vi "final_usrp_transceiver2.vi"() -> ()   [LabVIEW 2014]
uses:
  <vilib>/addons/Modulation/Analog/support/mod_Set Error Source.vi
  var_stop.vi
  <vilib>/addons/Modulation/Digital/Support/Common/Validators/mod_Generate Filter Coefficients Validate.vi
  <vilib>/addons/Modulation/Digital/General/subVIs/mod_Generate Filter Coefficients.vi
  <vilib>/measure/maspectr.llb/FFT Power Spectrum and PSD for 1 Chan (CDB).vi
  <vilib>/addons/Modulation/Digital/General/MT Apply Matched Filter (Generic).vi
  <vilib>/addons/Modulation/Digital/General/MT Align to Ideal Symbols (Generic).vi
  <instrlib>/niUSRP/niUSRP Fetch Rx Data (CDB Cluster).vi
  <instrlib>/niUSRP/niUSRP Write Tx Data (CDB Cluster).vi
  <vilib>/addons/Modulation/Digital/General/MT Apply Pulse Shaping Filter (Generic).vi
  <vilib>/addons/Modulation/niDMT.lvlib
  <vilib>/measure/NI_MAPro.lvlib
panel:
  in  "frame buffer size":i32=20
  in  "Stop":bool
  out "Frames Per Second":u32
  in  "energy threshold":dbl=-33.0 format="%#_13g"
  out "elements in frame buffer":i32
  out "valid frames":i32
  out "elements in send buffer":i32
  in  "packet size":i32=12800
  in  "Quality (0-1000)":i32=100 caption="Quality (750)"
  out "size(s) 4":i32
  out "frame num":u32
  out "length":i32[](array[numeric])
  out "start index":i32[](array[numeric])
  out "Numeric":i32
  out "size(s) 3":i32
  out "# elements in queue 2":i32
  out "size(s) 2":i32
  out "size(s)":i32[](array[numeric])
  out "image":T1(plugin-control)
  in  "Transmit power (db)":dbl
  out "found?":bool
  out "# elements in queue":i32
  out "valid?":bool
  in  "Gray code?":bool=TRUE
  in  "Modulation":enum16{"PSK", "QAM"}(ring)
  out "packet len":u32
  in  "filter length (symbols)":i32=8
  in  "filter parameter":dbl=0.5 format="%.2f"
  in  "pulse shaping filter (none)":T2(ring)=enum."Raised Cosine"
  in  "M-PSK (4)":i32=4 caption="M-ARY"
  in  "samples per symbol (16)":i32=4
  out "packet bits length":i32
  in  "number of samples":i64=40000
  out "RX coerced gain":dbl format="%#_6f"
  out "RX coerced carrier frequency":dbl=915000000.0 format="%#_6p"
  out "RX coerced IQ rate":dbl=4000000.0 format="%#_6p"
  in  "RX active antenna":string="RX2"
  in  "RX gain":dbl format="%#_6f"
  in  "RX device names":refnum<k15>="192.168.10.2"
  out "TX coerced gain":dbl format="%#_6f"
  out "TX coerced carrier frequency":dbl=915000000.0 format="%#_6p"
  out "coerced IQ rate":dbl=4000000.0 format="%#_6p"
  in  "TX device names":refnum<k15>="192.168.10.2"
  in  "TX gain":dbl format="%#_6f"
  in  "carrier frequency":dbl=915000000.0 format="%#_6p"
  in  "IQ rate":dbl=800000.0 format="%#_6p"
  in  "stop":bool
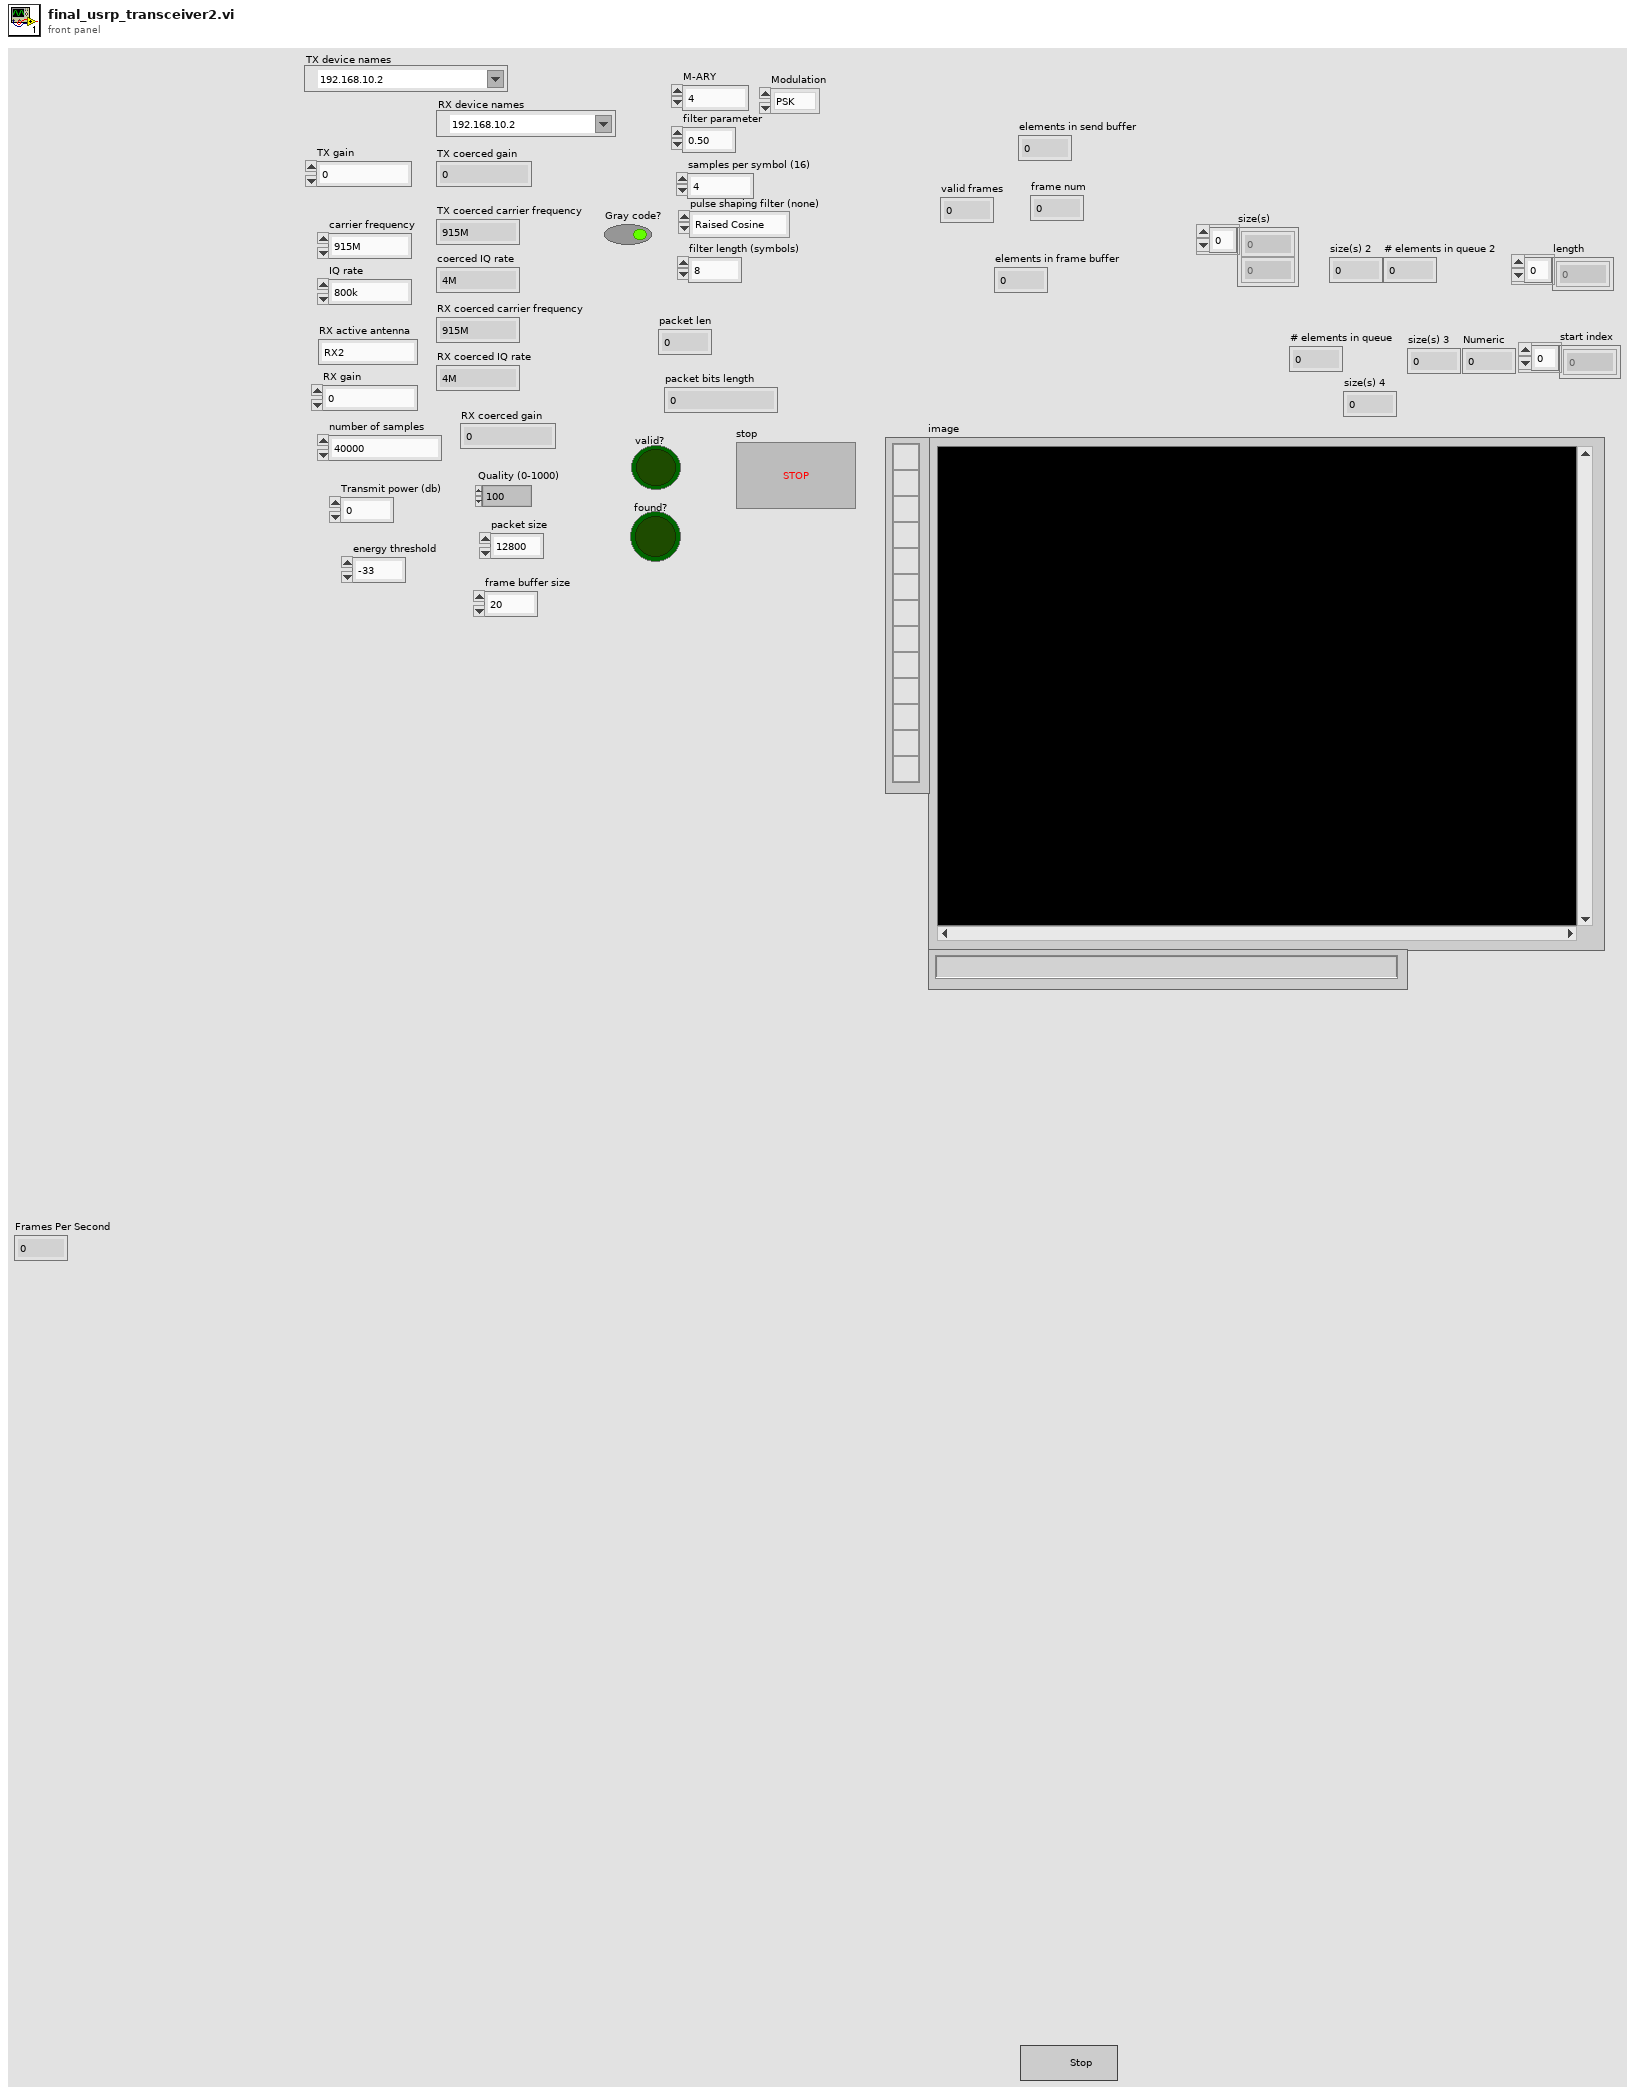
[diagram p1: front panel]
types:
  T1 = typedef "IMAQ Image.ctl" = refnum<image>
  T2 = enum16{"none", "Raised Cosine", "Root Raised Cos", "Gaussian"}
  T3 = enum16{"FSK", "PSK", "QAM", "MSK", "PAM", "ASK", "CPM"}
  T4 = cluster{"samples per symbol (16)":i32, "symbol map":cdb[], "index map":u32[]}
  T5 = cluster{"samples per symbol (16)":i32, "symbol map":cdb[], i32[]}
  T6 = typedef "IMAQ AVI2 Refnum.ctl" = refnum<k20>
  T7 = typedef "Image Type" = u32
  T8 = cluster{"Width":u32, "Height":u32, "Frames Per Second":u32, "Codec":string, "Has Data":bool}
  T9 = typedef "Semaphore RefNum" = refnum<k1>
  T10 = typedef "niAMT.lvlib/Complex Data Waveform.ctl" = cluster{"t0":dbl, "dt":dbl, "Y":cdb[]}
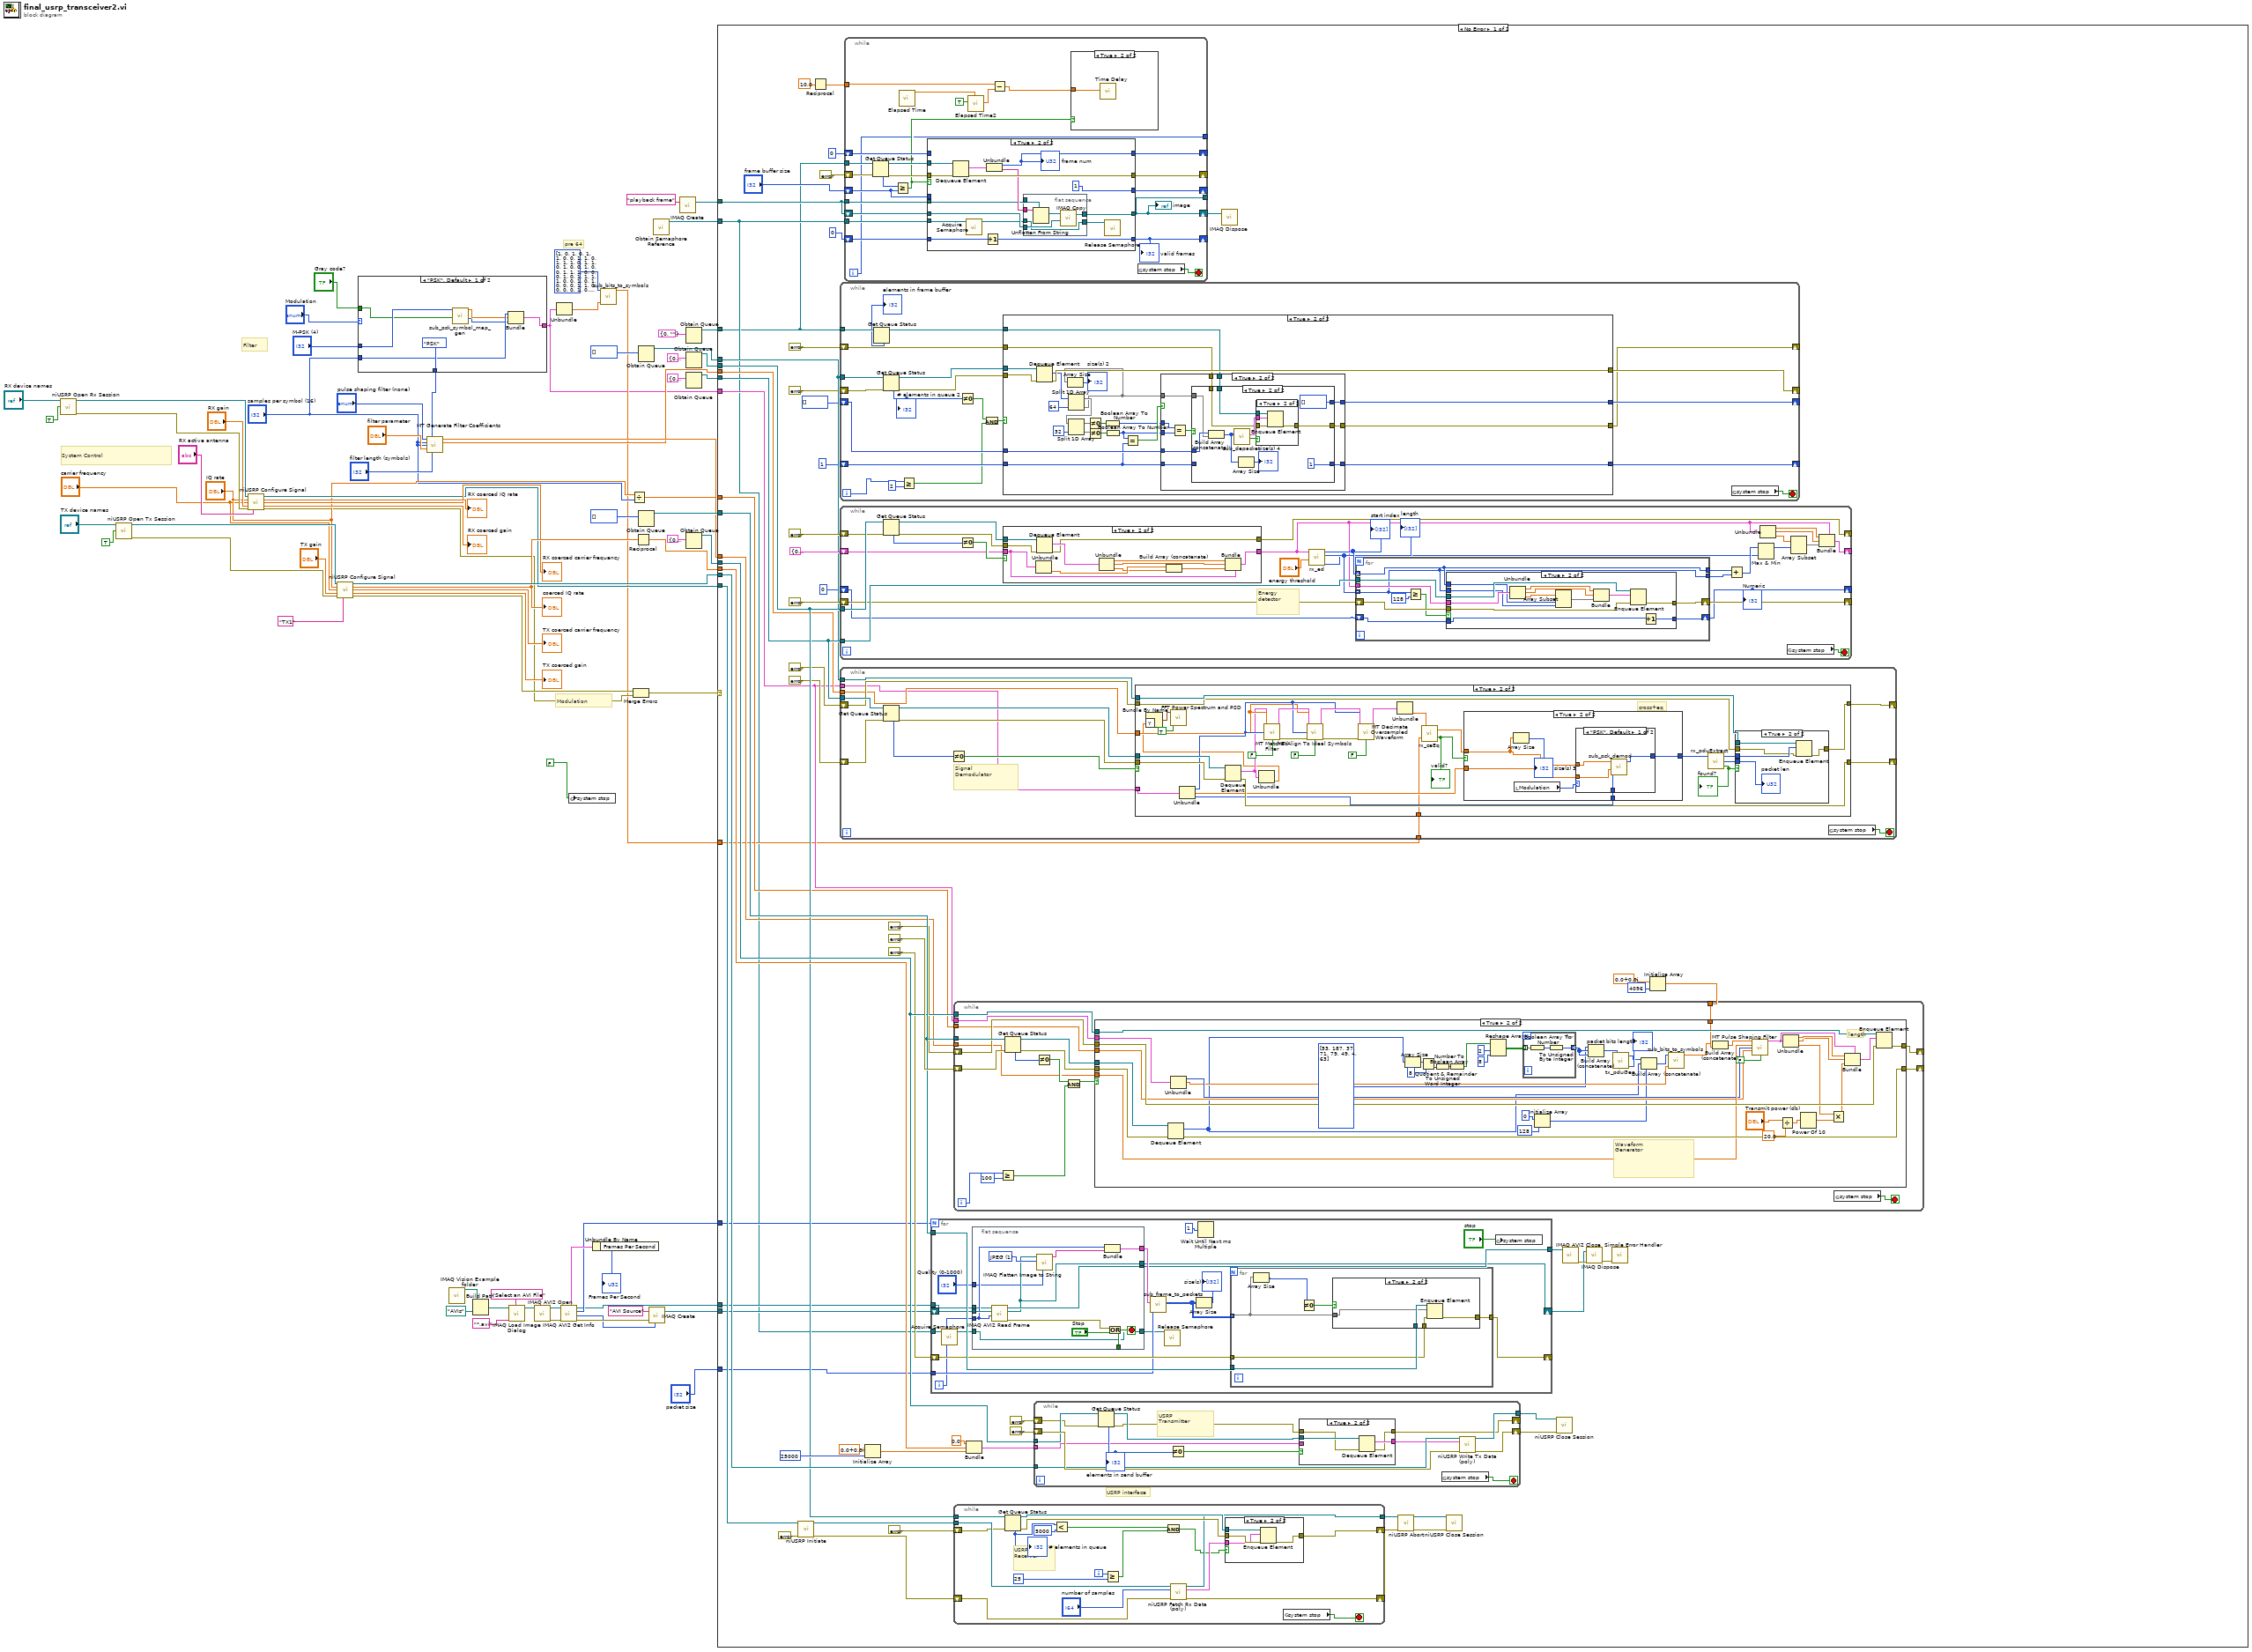
[diagram p0: block diagram]
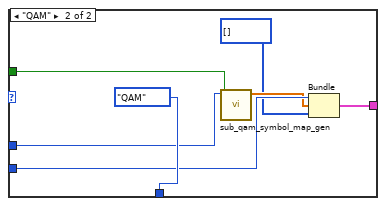
[diagram p2: hidden frame]
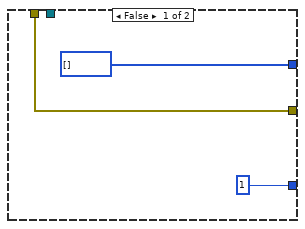
[diagram p7: hidden frame]
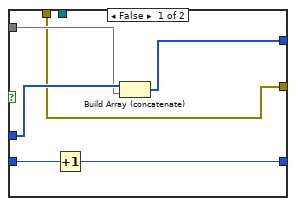
[diagram p8: hidden frame]
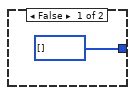
[diagram p11: hidden frame]
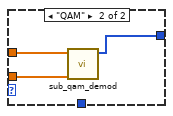
[diagram p12: hidden frame]
diagram:
  # "pre 64"
  # "Modulation"
  # "Filter"
  # "System Control"
  n1 = call <instrlib>:"niUSRP Open Rx Session.vi"("device names"="RX device names", "reset"=TRUE) -> ("session handle out"=w60:refnum<k15>, "error out"=w59:errorcluster)  [unwired: 12 in]
  n2 = call <instrlib>:"niUSRP Open Tx Session.vi"("device names"="TX device names", "reset"=TRUE) -> ("session handle out"=w73:refnum<k15>, "error out"=w72:errorcluster)  [unwired: 12 in]
  n3 = call <instrlib>:"niUSRP Configure Signal.vi"("session handle"=w60, "IQ rate"="IQ rate", "carrier frequency"="carrier frequency", "gain"="RX gain", "error in (no error)"=w59, "active antenna"="RX active antenna") -> ("session handle out"=w51:refnum<k15>, "coerced IQ rate"=→"RX coerced IQ rate":dbl, "coerced carrier frequency"=→"RX coerced carrier frequency":dbl, "coerced gain"=→"RX coerced gain":dbl, "error out"=w35:errorcluster)  [unwired: 5 in]
  n4 = call <instrlib>:"niUSRP Configure Signal.vi"("session handle"=w73, "IQ rate"="IQ rate", "carrier frequency"="carrier frequency", "gain"="TX gain", "error in (no error)"=w72, "active antenna"="TX1") -> ("session handle out"=w64:refnum<k15>, "coerced IQ rate"=w62:dbl, "coerced carrier frequency"=→"TX coerced carrier frequency":dbl, "coerced gain"=→"TX coerced gain":dbl, "error out"=w36:errorcluster)  [unwired: 5 in]
  "coerced IQ rate" <- w62
  n5 = case shown="\"PSK\", Default" "Modulation" {
    tunnel: [T3."PSK" ("modulation type") T3."QAM" ("modulation type")] -> w30
    tunnel: "M-PSK (4)" -> [w80 w86]
    tunnel: "Gray code?" -> [w79 w87]
    tunnel: "samples per symbol (16)" -> [w78 w85]
    tunnel: [w75 w82] -> w23
    frame "PSK", Default {
      n6 = call "sub_psk_symbol_map_gen.vi"("Gray code?"=w79, "M-PSK"=w80) -> ("index map"=w76:u32[], "symbol map"=w77:cdb[])  [unwired: 8 in]
      n7 = Bundle("samples per symbol (16)"=w78, "symbol map"=w77, "index map"=w76) -> (w75:T4)  [unwired: 1 in]
    }
    frame "QAM" {
      n8 = call "sub_qam_symbol_map_gen.vi"("Gray code?"=w87, "M-QAM"=w86) -> ("symbol map"=w84:cdb[])  [unwired: 9 in]
      n9 = Bundle("samples per symbol (16)"=w85, "symbol map"=w84, i32[] []) -> (w82:T5)  [unwired: 1 in]
    }
  }
  n10 = call <vilib>:"MT Generate Filter Coefficients.vi"("pulse shaping filter (none)"="pulse shaping filter (none)", "modulation type"=w30, "pulse shaping samples per symbol (16)"="samples per symbol (16)", "matched samples per symbol (16)"="samples per symbol (16)", "filter parameter"="filter parameter", "filter length (symbols)"="filter length (symbols)") -> ("pulse shaping filter coefficients"=w41:dbl[], "matched filter coefficients"=w39:dbl[])  [unwired: 7 in, 1 out]
  n11 = call "IMAQ Vision Example folder.vi"() -> ("Example Image Path"=w13:path)  [unwired: 11 in]
  n12 = Build Path(base path=w13, name or relative path=path "AVIs") -> (appended path=w10:path)
  n13 = call "IMAQ Load Image Dialog"("Prompt"="Select an AVI File" ("prompt"), "Pattern"="*.avi", "Start Path"=w10) -> ("Path"=w9:path)  [unwired: 6 in, 2 out]
  n14 = call "IMAQ AVI2 Open"("AVI File Path"=w9) -> ("error out"=w17:errorcluster, "AVI Refnum"=w16:T6)  [unwired: 2 in, 7 out]
  n15 = Unbundle(w23) -> ("symbol map"=w25:cdb[])  [unwired: 2 out]
  n16 = call "IMAQ AVI2 Get Info"("error in (no error)"=w17, "AVI Refnum"=w16) -> ("error out"=w15:errorcluster, "Image Type"=w14:T7, "Number of Frames"=w6:u32, "AVI Refnum (duplicate)"=w5:T6, "Frame Data"=w18:T8)  [unwired: 5 out]
  n17 = global write "var_stop.vi" "system stop"(FALSE) -> ()
  n18 = Unbundle By Name(w18) -> ("Frames Per Second"=→"Frames Per Second":u32)
  n19 = call "sub_bits_to_symbols.vi"("symbol map"=w25, "bits"=i16[] [1, 0, 1, 0, 1, 1, 0, 0, 1, 1, 0, 1, 1, 1, 0, 1, 1, 0, 1, 0, 0, 1, 0, 0, 1, 1, 1, 0, 0, 0, 1, 0, 1, 1, 1, 1, 0, 0, 1, 0, 1, 0, 0, 0, 1, 1, 0, 0, 0, 0, 1, 0, 0, 0, 0, 0, 1, 1, 1, 1, 1, 1, 0, 0] ("preamble(64) 2")) -> ("symbols"=w24:cdb[])  [unwired: 9 in]
  n20 = Divide(x="IQ rate", y="samples per symbol (16)") -> (x/y=w40:dbl)
  n21 = Merge Errors(w36, w35) -> (w34:errorcluster)
  n22 = Reciprocal(x=w62) -> (1/x=w61:dbl)
  n23 = Obtain Queue(element data type=i8[] [] ("output bit stream")) -> (queue out=w46:refnum<queue>)  [unwired: 4 in, 2 out]
  n24 = Obtain Queue(element data type=i16[] []) -> (queue out=w74:refnum<queue>)  [unwired: 4 in, 2 out]
  n25 = call "IMAQ Create"("Image Name"="AVI Source", "Image Type"=w14, "error in (no error)"=w15) -> ("New Image"=w4:T1)  [unwired: 1 in, 2 out]
  n26 = call <vilib>:"Obtain Semaphore Reference.vi"() -> ("semaphore"=w1:T9)  [unwired: 5 in, 2 out]
  n27 = call "IMAQ Create"("Image Name"="playback frame") -> ("New Image"=w2:T1)  [unwired: 3 in, 2 out]
  n28 = Obtain Queue(element data type=cluster{u32, "string":string} {0, "string"=""} ("frame")) -> (queue out=w21:refnum<queue>)  [unwired: 4 in, 2 out]
  n29 = Obtain Queue(element data type=cluster{"t0":dbl, "dt":dbl, "Y":cdb[]} {"t0"=0.0, "dt"=0.0, "Y"=[]} ("data")) -> (queue out=w50:refnum<queue>)  [unwired: 4 in, 2 out]
  n30 = Obtain Queue(element data type=cluster{"t0":dbl, "dt":dbl, "Y":cdb[]} {"t0"=0.0, "dt"=0.0, "Y"=[]} ("data")) -> (queue out=w47:refnum<queue>)  [unwired: 4 in, 2 out]
  n31 = Obtain Queue(element data type=cluster{"t0":dbl, "dt":dbl, "Y":cdb[]} {"t0"=0.0, "dt"=1.0, "Y"=[]} ("data")) -> (queue out=w65:refnum<queue>)  [unwired: 4 in, 2 out]
  n32 = case shown="No Error" w34 {
    tunnel: w74 -> [w151 _]
    tunnel: w65 -> [w146 _]
    tunnel: w64 -> [w147 _]
    tunnel: w61 -> [w140 _]
    tunnel: w51 -> [w135 _]
    tunnel: w50 -> [w129 _]
    tunnel: w47 -> [w125 _]
    tunnel: w46 -> [w123 _]
    tunnel: w23 -> [w117 _]
    tunnel: w41 -> [w120 _]
    tunnel: w40 -> [w119 _]
    tunnel: w39 -> [w118 _]
    tunnel: w24 -> [w111 _]
    tunnel: w21 -> [w89 _]
    tunnel: "packet size" -> [w102 _]
    tunnel: w6 -> [w99 _]
    tunnel: w5 -> [w98 _]
    tunnel: w4 -> [w97 _]
    tunnel: w2 -> [w91 _]
    tunnel: w1 -> [w90 _]
    frame No Error {
      # "USRP interface"
      n33 = call <instrlib>:"niUSRP Initiate.vi"("session handle"=w135, "error in (no error)"=errorcluster {"status"=FALSE, "code"=0, "source"=""}) -> ("session handle out"=w134:refnum<k15>, "error out"=w133:errorcluster)  [unwired: 12 in]
      n34 = Reciprocal(x=10.0) -> (1/x=w103:dbl)
      n35 = while {
        tunnel: w123 -> [w267]
        shift-right: [w260] -> _
        shift-left: errorcluster {"status"=FALSE, "code"=0, "source"=""} ("error out") -> [w266]
        shift-right: [w258] -> _
        shift-left: u32 1 -> [w259]
        shift-right: [w257] -> _
        shift-left: i8[] [] ("second subarray") -> [w256]
        tunnel: w89 -> [w255]
        shift-right: [w253] -> _
        shift-left: errorcluster {"status"=FALSE, "code"=0, "source"=""} ("error out") -> [w254]
        i -> [w251]
        stop <- w265 stop-if-true
        n36 = Get Queue Status(queue=w255) -> (queue out=w248:refnum<queue>, # elements in queue=→"elements in frame buffer":i32)  [unwired: 2 in, 6 out]
        n37 = Get Queue Status(queue=w267, error in (no error)=w266) -> (queue out=w262:refnum<queue>, error out=w261:errorcluster, # elements in queue=w264:i32)  [unwired: 1 in, 5 out]
        "# elements in queue 2" <- w264
        n38 = Greater Or Equal?(x=w251, y=2) -> (x >= y?=w250:bool)
        n39 = Not Equal To 0?(x=w264) -> (x != 0?=w263:bool)
        n40 = And(x=w263, y=w250) -> (x .and. y?=w249:bool)
        n41 = case shown="True" w249 {
          tunnel: w262 -> [_ w294]
          tunnel: w261 -> [w271 w293]
          tunnel: [w271 w292] -> w260
          tunnel: w259 -> [w270 w278]
          tunnel: [w270 w279] -> w258
          tunnel: [w268 w283] -> w257
          tunnel: w256 -> [w268 w280]
          tunnel: w248 -> [_ w277]
          tunnel: w254 -> [w269 w276]
          tunnel: [w269 w275] -> w253
          frame False {
          }
          frame True {
            n42 = Dequeue Element(queue=w294, error in (no error)=w293) -> (element=w274:i8[], error out=w292:errorcluster)  [unwired: 1 in, 2 out]
            n43 = Split 1D Array(array=w274, index=64) -> (first subarray=w285:i8[], second subarray=w272:i8[])
            n44 = Array Size(array=w272) -> (size(s)=→"size(s) 2":i32)
            n45 = Split 1D Array(array=w285, index=32) -> (first subarray=w288:i8[], second subarray=w289:i8[])
            n46 = Not Equal To 0?(x=w288) -> (x != 0?=w287:bool[])
            n47 = Not Equal To 0?(x=w289) -> (x != 0?=w286:bool[])
            n48 = Boolean Array To Number(Boolean array=w287) -> (number=w282:u32)
            n49 = Boolean Array To Number(Boolean array=w286) -> (number=w281:u32)
            n50 = Equal?(x=w281, y=w278) -> (x = y?=w284:bool)
            n51 = case shown="True" w284 {
              tunnel: [i8[] [] ("second subarray") w305] -> w283
              tunnel: w282 -> [_ w308]
              tunnel: w281 -> [_ w307]
              tunnel: w280 -> [_ w304]
              tunnel: w272 -> [_ w303]
              tunnel: [u32 1 w302] -> w279
              tunnel: w278 -> [_ w301]
              tunnel: w277 -> [_ w300]
              tunnel: w276 -> [w295 w299]
              tunnel: [w295 w298] -> w275
              frame False {
              }
              frame True {
                n52 = Equal?(x=w308, y=w307) -> (x = y?=w306:bool)
                n53 = case shown="True" w306 {
                  tunnel: [w312 i8[] [] ("second subarray")] -> w305
                  tunnel: w304 -> [w314 w323]
                  tunnel: w303 -> [w313 w322]
                  tunnel: [w310 u32 1] -> w302
                  tunnel: w301 -> [w311 _]
                  tunnel: w300 -> [_ w321]
                  tunnel: w299 -> [w309 w319]
                  tunnel: [w309 w318] -> w298
                  frame False {
                    n54 = Increment(x=w311) -> (x+1=w310:u32)
                    n55 = Build Array (concatenate)(w314, w313) -> (w312:i8[])
                  }
                  frame True {
                    n56 = Build Array (concatenate)(w323, w322) -> (w317:i8[])
                    n57 = call "sub_depacket.vi"("bitstream"=w317) -> ("CRC valid"=w315:bool, "frame"=w320:cluster{u32, "string":string})  [unwired: 9 in]
                    n58 = Array Size(array=w317) -> (size(s)=→"size(s) 4":i32)
                    n59 = case shown="True" w315 {
                      tunnel: w321 -> [_ w330]
                      tunnel: w320 -> [_ w329]
                      tunnel: w319 -> [w326 w328]
                      tunnel: [w326 w327] -> w318
                      frame False {
                      }
                      frame True {
                        n60 = Enqueue Element(queue=w330, element=w329, error in (no error)=w328) -> (error out=w327:errorcluster)  [unwired: 1 in, 2 out]
                      }
                    }
                  }
                }
              }
            }
          }
        }
        n61 = global read "var_stop.vi" "system stop"() -> (w265:bool)
      }
      n62 = while {
        tunnel: w129 -> [w425]
        shift-right: [w418] -> _
        shift-left: errorcluster {"status"=FALSE, "code"=0, "source"=""} ("error out") -> [w424]
        shift-right: [w404] -> _
        shift-left: cluster{"t0":dbl, "dt":dbl, "Y":cdb[]} {"t0"=0.0, "dt"=0.0, "Y"=[]} ("data") -> [w419]
        tunnel: w125 -> [w417]
        shift-right: [w416] -> _
        shift-left: errorcluster {"status"=FALSE, "code"=0, "source"=""} ("error out") -> [w415]
        shift-right: [w399] -> _
        shift-left: 0 -> [w400]
        stop <- w414 stop-if-true
        # "Energy\ndetector"
        n63 = Get Queue Status(queue=w425, error in (no error)=w424) -> (queue out=w420:refnum<queue>, error out=w421:errorcluster, # elements in queue=w423:i32)  [unwired: 1 in, 5 out]
        n64 = Not Equal To 0?(x=w423) -> (x != 0?=w422:bool)
        n65 = case shown="True" w422 {
          tunnel: w421 -> [w452 w463]
          tunnel: w420 -> [_ w462]
          tunnel: w419 -> [w451 w457]
          tunnel: [w452 w454] -> w418
          tunnel: [w451 w453] -> w411
          frame False {
          }
          frame True {
            n66 = Unbundle(w457) -> ("Y"=w460:cdb[])  [unwired: 2 out]
            n67 = Dequeue Element(queue=w462, error in (no error)=w463) -> (element=w461:cluster{"t0":dbl, "dt":dbl, "Y":cdb[]}, error out=w454:errorcluster)  [unwired: 1 in, 2 out]
            n68 = Unbundle(w461) -> ("t0"=w456:dbl, "dt"=w455:dbl, "Y"=w459:cdb[])
            n69 = Build Array (concatenate)(w460, w459) -> (w458:cdb[])
            n70 = Bundle(cluster=w457, "t0"=w456, "dt"=w455, "Y"=w458) -> (w453:cluster{"t0":dbl, "dt":dbl, "Y":cdb[]})
          }
        }
        n71 = call "rx_ed.vi"("energy threshold"="energy threshold", "Wavefrom"=w411) -> ("first pulse"=w401:i32, "length"=w412:i32[], "start index"=w413:i32[])  [unwired: 7 in]
        "start index" <- w413
        "length" <- w412
        n72 = for {
          tunnel: w417 -> [w435]
          tunnel: w411 -> [w432]
          shift-right: [w434] -> w416
          shift-left: w415 -> [w433]
          tunnel: w413 -> [w431] mode=indexing
          tunnel: w412 -> [w430] mode=indexing
          tunnel: [w431] -> w407
          tunnel: [w430] -> w406
          shift-right: [w426] -> w399
          shift-left: w400 -> [w427]
          n73 = Greater Or Equal?(x=w430, y=128) -> (x >= y?=w428:bool)
          n74 = case shown="True" w428 {
            tunnel: w435 -> [_ w450]
            tunnel: [w437 w449] -> w434
            tunnel: w433 -> [w437 w448]
            tunnel: w432 -> [_ w447]
            tunnel: w431 -> [_ w441]
            tunnel: w430 -> [_ w440]
            tunnel: w427 -> [w436 w439]
            tunnel: [w436 w438] -> w426
            frame False {
            }
            frame True {
              n75 = Unbundle(w447) -> ("t0"=w445:dbl, "dt"=w446:dbl, "Y"=w443:cdb[])
              n76 = Array Subset(array=w443, index=w441, length=w440) -> (w442:cdb[])
              n77 = Bundle("t0"=w445, "dt"=w446, w442) -> (w444:cluster{"t0":dbl, "dt":dbl, cdb[]})  [unwired: 1 in]
              n78 = Enqueue Element(queue=w450, element=w444, error in (no error)=w448) -> (error out=w449:errorcluster)  [unwired: 1 in, 2 out]
              n79 = Increment(x=w439) -> (x+1=w438:i32)
            }
          }
        }
        "Numeric" <- w399
        n80 = Add(x=w407, y=w406) -> (x+y=w403:i32)
        n81 = Max & Min(x=w403, y=w401) -> (max(x,y)=w402:i32)  [unwired: 1 out]
        n82 = Unbundle(w411) -> ("t0"=w410:dbl, "dt"=w409:dbl, "Y"=w408:cdb[])
        n83 = global read "var_stop.vi" "system stop"() -> (w414:bool)
        n84 = Array Subset(array=w408, index=w402) -> (w405:cdb[])  [unwired: 1 in]
        n85 = Bundle(cluster=w411, "t0"=w410, "dt"=w409, "Y"=w405) -> (w404:cluster{"t0":dbl, "dt":dbl, "Y":cdb[]})
      }
      n86 = while {
        tunnel: w125 -> [w344]
        shift-right: [w338] -> _
        shift-left: errorcluster {"status"=FALSE, "code"=0, "source"=""} ("error out") -> [w343]
        tunnel: w123 -> [w337]
        shift-right: [w336] -> _
        shift-left: errorcluster {"status"=FALSE, "code"=0, "source"=""} ("error out") -> [w335]
        tunnel: w118 -> [w333]
        tunnel: w117 -> [w332]
        tunnel: w111 -> [w331]
        stop <- w334 stop-if-true
        # "Signal \nDemodulator"
        n87 = Get Queue Status(queue=w344, error in (no error)=w343) -> (queue out=w340:refnum<queue>, error out=w339:errorcluster, # elements in queue=w342:i32)  [unwired: 1 in, 5 out]
        n88 = Not Equal To 0?(x=w342) -> (x != 0?=w341:bool)
        n89 = case shown="True" w341 {
          tunnel: w340 -> [_ w376]
          tunnel: w339 -> [w346 w377]
          tunnel: [w346 w375] -> w338
          tunnel: w337 -> [_ w365]
          tunnel: [w345 w364] -> w336
          tunnel: w335 -> [w345 w363]
          tunnel: w333 -> [_ w352]
          tunnel: w332 -> [_ w356]
          tunnel: w331 -> [_ w349]
          frame False {
          }
          frame True {
            # "cross+eq"
            n90 = Unbundle(w356) -> ("samples per symbol (16)"=w355:i32, "symbol map"=w354:cdb[], "index map"=w353:u32[])
            n91 = Dequeue Element(queue=w376, error in (no error)=w377) -> (element=w348:cluster{"t0":dbl, "dt":dbl, "Y":cdb[]}, error out=w375:errorcluster)  [unwired: 1 in, 2 out]
            n92 = Unbundle(w348) -> ("Y"=w347:cdb[])  [unwired: 2 out]
            n93 = Bundle By Name("Y"=w347) -> (w351:waveform(cdb))  [unwired: 1 in]
            n94 = call-poly <vilib>:"FFT Power Spectrum and PSD.vi"("dB On (F)"=TRUE, "time signal"=w351) -> ()  [unwired: 6 in, 4 out]
            n95 = call-poly <vilib>:"MT Matched Filter.vi"("input complex waveform"=w348, "matched filter coefficients"=w352, "samples per symbol (16)"=w355, "reset? (T)"=FALSE) -> ("output complex waveform"=w374:T10, "error out"=w373:errorcluster)  [unwired: 10 in]
            n96 = call-poly <vilib>:"MT Align To Ideal Symbols.vi"("input complex waveform"=w374, "matched filter coefficients"=w352, "samples per symbol (16)"=w355, "error in (no error)"=w373, "reset? (T)"=FALSE) -> ("output complex waveform"=w371:T10, "error out"=w372:errorcluster)  [unwired: 8 in, 1 out]
            n97 = call <vilib>:"MT Decimate Oversampled Waveform.vi"("input complex waveform"=w371, "decimation factor"=w355, "error in (no error)"=w372, "reset? (T)"=FALSE) -> ("output complex waveform"=w370:T10)  [unwired: 10 in, 1 out]
            n98 = Unbundle(w370) -> ("Y"=w366:cdb[])  [unwired: 2 out]
            n99 = call "rx_ceEq.vi"("preamble"=w349, "symbols"=w366) -> ("valid?"=w361:bool, "eq symbols"=w362:cdb[])
            "valid?" <- w361
            n100 = case shown="True" w361 {
              tunnel: [i8[] [] ("output bit stream") w382] -> w369
              tunnel: w354 -> [_ w383]
              tunnel: w362 -> [_ w380]
              tunnel: w353 -> [_ w381]
              frame False {
              }
              frame True {
                n101 = Array Size(array=w380) -> (size(s)=→"size(s) 3":i32)
                n102 = local read "Modulation"() -> (w384:enum16{"PSK", "QAM"})
                n103 = case shown="\"PSK\", Default" w384 {
                  tunnel: w380 -> [w388 w391]
                  tunnel: w383 -> [w387 w390]
                  tunnel: [w385 w389] -> w382
                  tunnel: w381 -> [w386 _]
                  frame "PSK", Default {
                    n104 = call "sub_psk_demod.vi"("index map"=w386, "symbol map"=w387, "symbol"=w388) -> ("bitstream"=w385:i16[])  [unwired: 8 in]
                  }
                  frame "QAM" {
                    n105 = call "sub_qam_demod.vi"("symbol map"=w390, "symbol"=w391) -> ("bitstream"=w389:i16[])  [unwired: 9 in]
                  }
                }
              }
            }
            n106 = call "rx_pduExtract.vi"("output bit stream"=w369) -> ("found?"=w368:bool, "packet len"=w360:u32, "ppdu"=w367:i8[])  [unwired: 2 in]
            "found?" <- w368
            n107 = case shown="True" w368 {
              tunnel: w367 -> [_ w395]
              tunnel: w365 -> [_ w397]
              tunnel: [w392 w396] -> w364
              tunnel: w363 -> [w392 w393]
              tunnel: w360 -> [_ w394]
              frame False {
              }
              frame True {
                n108 = Enqueue Element(queue=w397, element=w395, error in (no error)=w393) -> (error out=w396:errorcluster)  [unwired: 1 in, 2 out]
                "packet len" <- w394
              }
            }
          }
        }
        n109 = global read "var_stop.vi" "system stop"() -> (w334:bool)
      }
      n110 = while {
        tunnel: w89 -> [w219]
        shift-right: [w215] -> _
        shift-left: errorcluster {"status"=FALSE, "code"=0, "source"=""} ("error out") -> [w218]
        shift-right: [w212] -> _
        shift-left: 0 -> [w211]
        tunnel: w103 -> [w207]
        shift-right: [w208] -> _
        shift-left: 0 -> [w209]
        shift-right: [w203] -> _
        shift-left: "frame buffer size" -> [w202]
        shift-right: [w196] -> w92
        shift-left: w91 -> [w200]
        tunnel: w91 -> [w199]
        tunnel: w90 -> [w198]
        tunnel: [w197] -> _
        tunnel: [w196] -> _
        i -> [w197]
        stop <- w214 stop-if-true
        n111 = Get Queue Status(queue=w219, error in (no error)=w218) -> (queue out=w217:refnum<queue>, error out=w216:errorcluster, # elements in queue=w204:i32)  [unwired: 1 in, 5 out]
        n112 = Greater Or Equal?(x=w204, y=w202) -> (x >= y?=w201:bool)
        n113 = call "Elapsed Time"() -> ("Present (s)"=w206:dbl)  [unwired: 12 in, 7 out]
        n114 = case shown="True" w201 {
          tunnel: w217 -> [_ w240]
          tunnel: w216 -> [w225 w239]
          tunnel: [w225 w237] -> w215
          tunnel: [w224 w235] -> w212
          tunnel: w211 -> [w224 _]
          tunnel: w209 -> [w223 w234]
          tunnel: [w223 w233] -> w208
          tunnel: [w222 1] -> w203
          tunnel: w202 -> [w222 _]
          tunnel: [w221 w230] -> w196
          tunnel: w200 -> [w221 w229]
          tunnel: w199 -> [_ w231]
          tunnel: w198 -> [_ w228]
          frame False {
          }
          frame True {
            n115 = Dequeue Element(queue=w240, error in (no error)=w239) -> (element=w238:cluster{u32, "string":string}, error out=w237:errorcluster)  [unwired: 1 in, 2 out]
            n116 = call <vilib>:"Acquire Semaphore.vi"("semaphore"=w228) -> ("semaphore out"=w227:T9)  [unwired: 4 in, 2 out]
            n117 = Increment(x=w234) -> (x+1=w233:i32)
            n118 = Unbundle(w238) -> (w235:u32, "string"=w236:string)
            "frame num" <- w235
            n119 = flat-sequence {
              tunnel: w236 -> [w246]
              tunnel: w231 -> [w245]
              tunnel: [w243] -> w230
              tunnel: w229 -> [w242]
              tunnel: w227 -> [w241]
              tunnel: [w241] -> w226
              frame #0 {
                n120 = Unflatten From String(type=w245, binary string=w246) -> (value=w244:T1)  [unwired: 3 in, 2 out]
                n121 = call "IMAQ Copy"("Image Dst"=w242, "Image Src"=w244) -> ("Image Dst Out"=w243:T1)  [unwired: 4 in, 1 out]
              }
            }
            n122 = call <vilib>:"Release Semaphore.vi"("semaphore"=w226) -> ()  [unwired: 5 in, 2 out]
          }
        }
        "valid frames" <- w208
        "image" <- w196
        n123 = call "Elapsed Time2"("Reset"=TRUE, "Set Start Time (s)"=w206) -> ("Elapsed Time (s)"=w210:dbl)  [unwired: 10 in, 7 out]
        n124 = Subtract(x=w207, y=w210) -> (x-y=w205:dbl)
        n125 = case shown="True" w201 {
          tunnel: w205 -> [_ w220]
          frame False {
          }
          frame True {
            n126 = call "Time Delay"("Delay Time (s)"=w220) -> ()  [unwired: 10 in, 1 out]
          }
        }
        n127 = global read "var_stop.vi" "system stop"() -> (w214:bool)
      }
      n128 = Initialize Array(cdb 0.0+0.0i, 25000 ("dimension size")) -> (w141:cdb[])
      n129 = for {
        N: w99 -> [_]
        tunnel: w151 -> [w170]
        shift-right: [w168] -> _
        shift-left: errorcluster {"status"=FALSE, "code"=0, "source"=""} ("error out") -> [w169]
        tunnel: w102 -> [w164]
        tunnel: w98 -> [w160]
        tunnel: [w159] -> w94
        shift-right: [w158] -> w93
        shift-left: w97 -> [w163]
        tunnel: w90 -> [w155]
        i -> [w162]
        stop <- w157 stop-if-true
        n130 = call <vilib>:"Acquire Semaphore.vi"("semaphore"=w155) -> ("semaphore out"=w154:T9)  [unwired: 4 in, 2 out]
        n131 = flat-sequence {
          tunnel: w163 -> [w180]
          tunnel: w162 -> [w179]
          tunnel: [w178] -> w161
          tunnel: w160 -> [w177]
          tunnel: [w176] -> w159
          tunnel: [w175] -> w158
          tunnel: [w174] -> w157
          tunnel: "Quality (0-1000)" -> [w173]
          tunnel: w154 -> [w172]
          tunnel: [w172] -> w153
          frame #0 {
            w182 = 1 items=["None", "JPEG", "PACKED BINARY"] ("Compression (None)")
            n132 = call "IMAQ AVI2 Read Frame"("Frame Number"=w179, "Image"=w180, "AVI Refnum"=w177) -> ("error out"=w183:errorcluster, "Image Out"=w175:T1, "AVI Refnum (duplicate)"=w176:T6)  [unwired: 1 in, 5 out]
            n133 = call "IMAQ Flatten Image to String"("Quality (750)"=w173, "Compression (None)"=w182, "Image"=w175) -> ("Data String"=w181:string)  [unwired: 7 in, 1 out]
            n134 = Bundle(w179, "Data String"=w181) -> (w178:cluster{i32, "Data String":string})  [unwired: 1 in]
            n135 = Or(x=w183, y="Stop") -> (x .or. y?=w174:bool)
          }
        }
        n136 = call "sub_frame_to_packets.vi"("packet size"=w164, "Cluster"=w161) -> ("packets"=w167:i16[][])  [unwired: 9 in]
        n137 = call <vilib>:"Release Semaphore.vi"("semaphore"=w153) -> ()  [unwired: 5 in, 2 out]
        n138 = Array Size(array=w167) -> (size(s)=→"size(s)":i32[])
        n139 = Wait Until Next ms Multiple(millisecond multiple=u32 1) -> ()  [unwired: 1 out]
        n140 = for {
          tunnel: w170 -> [w190]
          tunnel: w169 -> [w189]
          tunnel: [w188] -> w168
          tunnel: w167 -> [w185] mode=indexing
          n141 = Array Size(array=w185) -> (size(s)=w186:i32)
          n142 = Not Equal To 0?(x=w186) -> (x != 0?=w187:bool)
          n143 = case shown="True" w187 {
            tunnel: w185 -> [_ w192]
            tunnel: w190 -> [_ w195]
            tunnel: w189 -> [w191 w194]
            tunnel: [w191 w193] -> w188
            frame False {
            }
            frame True {
              n144 = Enqueue Element(queue=w195, element=w192, error in (no error)=w194) -> (error out=w193:errorcluster)  [unwired: 1 in, 2 out]
            }
          }
        }
        n145 = global write "var_stop.vi" "system stop"("stop") -> ()
      }
      n146 = while {
        tunnel: w134 -> [w482]
        shift-right: [w471] -> w130
        shift-left: w133 -> [w481]
        tunnel: w129 -> [w479]
        shift-right: [w473] -> _
        shift-left: errorcluster {"status"=FALSE, "code"=0, "source"=""} ("error out") -> [w478]
        tunnel: [w472] -> w131
        i -> [w469]
        stop <- w470 stop-if-true
        # "USRP\nReceiver"
        n147 = Get Queue Status(queue=w479, error in (no error)=w478) -> (queue out=w475:refnum<queue>, error out=w474:errorcluster, # elements in queue=w477:i32)  [unwired: 1 in, 5 out]
        "# elements in queue" <- w477
        n148 = Less?(x=w477, y=5000) -> (x < y?=w467:bool)
        n149 = Greater Or Equal?(x=w469, y=25) -> (x >= y?=w466:bool)
        n150 = And(x=w467, y=w466) -> (x .and. y?=w464:bool)
        n151 = call-poly <instrlib>:"niUSRP Fetch Rx Data (poly).vi"("session handle"=w482, "number of samples"="number of samples", "error in (no error)"=w481) -> ("session handle out"=w472:refnum<k15>, "data"=w465:cluster{"t0":dbl, "dt":dbl, "Y":cdb[]}, "error out"=w471:errorcluster)  [unwired: 9 in, 1 out]
        n152 = case shown="True" w464 {
          tunnel: w475 -> [_ w487]
          tunnel: w474 -> [w483 w486]
          tunnel: [w483 w485] -> w473
          tunnel: w465 -> [_ w484]
          frame False {
          }
          frame True {
            n153 = Enqueue Element(queue=w487, element=w484, error in (no error)=w486) -> (error out=w485:errorcluster)  [unwired: 1 in, 2 out]
          }
        }
        n154 = global read "var_stop.vi" "system stop"() -> (w470:bool)
      }
      n155 = Bundle(0.0, w140, w141) -> (w138:cluster{dbl, dbl, cdb[]})  [unwired: 1 in]
      n156 = while {
        shift-right: [w497] -> w150
        shift-left: errorcluster {"status"=FALSE, "code"=0, "source"=""} ("error out") -> [w495]
        tunnel: [w496] -> w149
        tunnel: w147 -> [w494]
        tunnel: w146 -> [w492]
        shift-right: [w490] -> _
        shift-left: errorcluster {"status"=FALSE, "code"=0, "source"=""} ("error out") -> [w491]
        tunnel: w138 -> [w489]
        stop <- w488 stop-if-true
        # "USRP\nTransmitter"
        n157 = Get Queue Status(queue=w492, error in (no error)=w491) -> (queue out=w499:refnum<queue>, error out=w498:errorcluster, # elements in queue=w501:i32)  [unwired: 1 in, 5 out]
        "elements in send buffer" <- w501
        n158 = Not Equal To 0?(x=w501) -> (x != 0?=w500:bool)
        n159 = case shown="True" w500 {
          tunnel: w499 -> [_ w507]
          tunnel: w498 -> [w502 w506]
          tunnel: [w503 w505] -> w493
          tunnel: [w502 w504] -> w490
          tunnel: w489 -> [w503 _]
          frame False {
          }
          frame True {
            n160 = Dequeue Element(queue=w507, error in (no error)=w506) -> (element=w505:cluster{"t0":dbl, "dt":dbl, "Y":cdb[]}, error out=w504:errorcluster)  [unwired: 1 in, 2 out]
          }
        }
        n161 = global read "var_stop.vi" "system stop"() -> (w488:bool)
        n162 = call-poly <instrlib>:"niUSRP Write Tx Data (poly).vi"("session handle"=w494, "data"=w493, "error in (no error)"=w495) -> ("session handle out"=w496:refnum<k15>, "error out"=w497:errorcluster)  [unwired: 11 in]
      }
      n163 = call "IMAQ Dispose"("Image"=w92) -> ()  [unwired: 2 in, 4 out]
      n164 = call <instrlib>:"niUSRP Abort.vi"("session handle"=w131, "error in (no error)"=w130) -> ("session handle out"=w137:refnum<k15>, "error out"=w136:errorcluster)  [unwired: 12 in]
      n165 = call <instrlib>:"niUSRP Close Session.vi"("session handle"=w137, "error in (no error)"=w136) -> ()  [unwired: 13 in, 1 out]
      n166 = call <instrlib>:"niUSRP Close Session.vi"("session handle"=w149, "error in (no error)"=w150) -> ()  [unwired: 13 in, 1 out]
      n167 = call "IMAQ AVI2 Close"("AVI Refnum"=w94) -> ("error out"=w95:errorcluster)  [unwired: 1 in, 9 out]
      n168 = call "IMAQ Dispose"("Image"=w93, "error in (no error)"=w95) -> ("error out"=w96:errorcluster)  [unwired: 1 in, 3 out]
      n169 = call <vilib>:"Simple Error Handler.vi"("error in (no error)"=w96) -> ()  [unwired: 1 in, 8 out]
      n170 = Initialize Array(cdb 0.0+0.0i, 4096 ("dimension size")) -> (w112:cdb[])
      n171 = while {
        tunnel: w151 -> [w523]
        shift-right: [w520] -> _
        shift-left: errorcluster {"status"=FALSE, "code"=0, "source"=""} ("error out") -> [w526]
        tunnel: w146 -> [w519]
        shift-right: [w518] -> _
        shift-left: errorcluster {"status"=FALSE, "code"=0, "source"=""} ("error out") -> [w517]
        tunnel: w117 -> [w515]
        tunnel: w120 -> [w514]
        tunnel: w119 -> [w513]
        tunnel: w112 -> [w512]
        i -> [w511]
        stop <- w516 stop-if-true
        n172 = Greater Or Equal?(x=w511, y=100) -> (x >= y?=w508:bool)
        n173 = Get Queue Status(queue=w523, error in (no error)=w526) -> (queue out=w521:refnum<queue>, error out=w522:errorcluster, # elements in queue=w525:i32)  [unwired: 1 in, 5 out]
        n174 = Not Equal To 0?(x=w525) -> (x != 0?=w524:bool)
        n175 = And(x=w524, y=w508) -> (x .and. y?=w509:bool)
        n176 = case shown="True" w509 {
          tunnel: w522 -> [w528 w571]
          tunnel: w521 -> [_ w570]
          tunnel: [w528 w569] -> w520
          tunnel: w519 -> [_ w564]
          tunnel: [w527 w563] -> w518
          tunnel: w517 -> [w527 w562]
          tunnel: w515 -> [_ w559]
          tunnel: w514 -> [_ w558]
          tunnel: w513 -> [_ w557]
          tunnel: w512 -> [_ w547]
          frame False {
          }
          frame True {
            # "length"
            # "Waveform \nGenerator"
            n177 = Dequeue Element(queue=w570, error in (no error)=w571) -> (element=w531:i16[], error out=w569:errorcluster)  [unwired: 1 in, 2 out]
            n178 = Unbundle(w559) -> ("samples per symbol (16)"=w553:i32, "symbol map"=w546:cdb[])  [unwired: 1 out]
            n179 = Array Size(array=w531) -> (size(s)=w555:i32)
            n180 = Quotient & Remainder(x=w555, y=8) -> (floor(x/y)=w535:i32)  [unwired: 1 out]
            n181 = To Unsigned Word Integer(number=w535) -> (unsigned 16bit integer=w554:u16)
            n182 = Number To Boolean Array(number=w554) -> (Boolean array=w568:bool[])
            n183 = Reshape Array(w568, 2 ("dimension size"), 8 ("dimension size")) -> (w565:bool[][])
            n184 = for {
              tunnel: w565 -> [w574] mode=indexing
              tunnel: [w572] -> w556 mode=indexing
              n185 = Boolean Array To Number(Boolean array=w574) -> (number=w573:u32)
              n186 = To Unsigned Byte Integer(number=w573) -> (unsigned 8bit integer=w572:u8)
            }
            n187 = Initialize Array(u8 0, 128 ("dimension size")) -> (w530:u8[])
            n188 = Build Array (concatenate)(u8[] [53, 187, 37, 71, 79, 49, 4, 63] ("Array 2"), w556, w556) -> (w561:u8[])
            n189 = call "tx_pduGen.vi"("byte array"=w561) -> ("packet bits length"=→"packet bits length":i32, "pdu"=w532:i32[])  [unwired: 3 in]
            n190 = Build Array (concatenate)(w532, w531, w530) -> (w529:i32[])
            n191 = call "sub_bits_to_symbols.vi"("symbol map"=w546, "bits"=w529) -> ("symbols"=w545:cdb[])  [unwired: 9 in]
            n192 = Build Array (concatenate)(w545, w547) -> (w543:cdb[])
            n193 = call-poly <vilib>:"MT Pulse Shaping Filter.vi"("symbols"=w543, "pulse shaping filter coefficients"=w558, "samples per symbol (16)"=w553, "symbol rate (Hz)"=w557, "reset? (T)"=FALSE) -> ("output complex waveform"=w552:T10)  [unwired: 9 in, 1 out]
            n194 = Divide(x="Transmit power (db)", y=20.0) -> (x/y=w540:dbl)
            n195 = Unbundle(w552) -> ("t0"=w551:dbl, "dt"=w550:dbl, "Y"=w538:cdb[])
            n196 = Power Of 10(x=w540) -> (10^x=w539:dbl)
            n197 = Multiply(x=w538, y=w539) -> (x*y=w537:cdb[])
            n198 = Bundle(cluster=w552, "t0"=w551, "dt"=w550, "Y"=w537) -> (w549:T10)
            n199 = Enqueue Element(queue=w564, element=w549, error in (no error)=w562) -> (error out=w563:errorcluster)  [unwired: 1 in, 2 out]
          }
        }
        n200 = global read "var_stop.vi" "system stop"() -> (w516:bool)
      }
    }
    frame Error {
    }
  }
